vi "Acquire Data from Hardware N times.vi"(10 "User Specified":T1={"Hardware Configuration"={"Signal Channel"="PXI1Slot7/ao0", "Response Channel"="PXI1Slot7/ai0", "Trigger Channel"="/PXI1Slot7/PFI0", "Number of Acquisitions"=1.0}, "Analysis Configuration"={"Statistics"=TRUE}, "Signal Type"=enum."From Excel", "New Data Behavior"=enum."Replace", "Signal Configuration"={"Chirp Amplitude"=0.0, "I/O Limit"=0.0, "Sample Rate"=0.0, "Chirp Duration (s)"=0.0, "Upper Frequency"=0.0, "Lower Frequency"=0.0, "Windowing"=enum."None"}, "Waveform File"="", "Save Location"=""}) -> (0 "error out":errorcluster)   [LabVIEW 2017]
doc: "Generates sample waveforms according to the signal type in the HW Config input."
uses:
  controls/User Specified Data.ctl
  controls/HW Configuration.ctl
  controls/Analysis Configuration.ctl
  controls/New Data Behavior.ctl
  controls/Signal Configuration.ctl
  <vilib>/DAQmx/write.llb/DAQmx Write (Analog Wfm 1Chan NSamp).vi
  <vilib>/DAQmx/read.llb/DAQmx Read (Analog Wfm 1Chan NSamp).vi
  <vilib>/DAQmx/create/channels.llb/DAQmx Create Channel (AO-Voltage-Basic).vi
  <vilib>/DAQmx/configure/timing.llb/DAQmx Timing (Sample Clock).vi
  <vilib>/DAQmx/configure/trigger.llb/DAQmx Start Trigger (Digital Edge).vi
  <vilib>/DAQmx/miscellaneous.llb/DAQmx Fill In Error Info.vi
  <vilib>/DAQmx/create/channels.llb/DAQmx Create Channel (AI-Voltage-Basic).vi
  <vilib>/DAQmx/configure/task.llb/DAQmx Configure Logging (TDMS).vi
panel:
  in  "error in":errorcluster
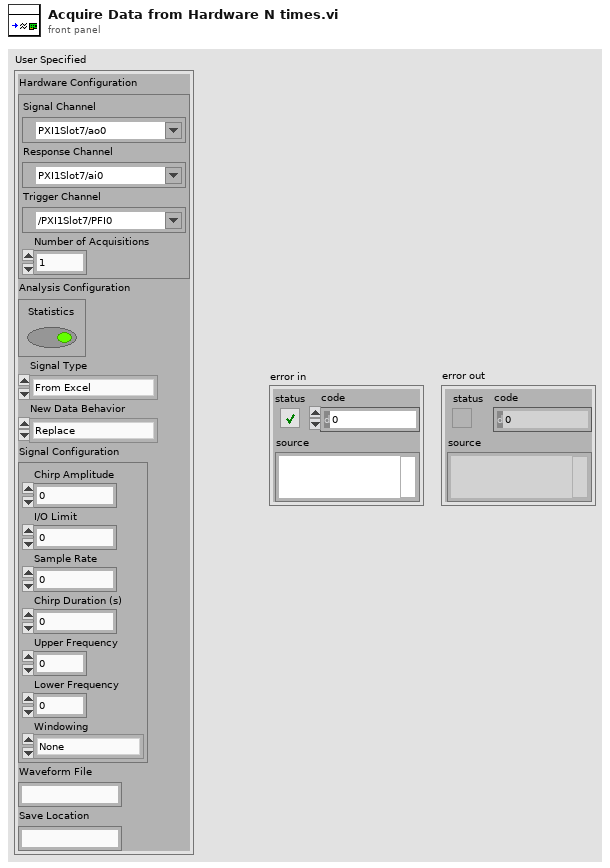
[diagram p1: front panel]
types:
  T1 = typedef "User Specified Data.ctl" = cluster{"Hardware Configuration":T2, "Analysis Configuration":T3, "Signal Type":enum16{"From Excel", "Single Chirp"}, "New Data Behavior":T4, "Signal Configuration":T5, "Waveform File":string, "Save Location":string}
  T2 = typedef "HW Configuration.ctl" = cluster{"Signal Channel":tag, "Response Channel":tag, "Trigger Channel":tag, "Number of Acquisitions":dbl}
  T3 = typedef "Analysis Configuration.ctl" = cluster{"Statistics":bool}
  T4 = typedef "New Data Behavior.ctl" = enum16{"Replace", "Overlay", "Append"}
  T5 = typedef "Signal Configuration.ctl" = cluster{"Chirp Amplitude":dbl, "I/O Limit":dbl, "Sample Rate":dbl, "Chirp Duration (s)":dbl, "Upper Frequency":dbl, "Lower Frequency":dbl, "Windowing":enum16{"None", "Exponential", "Flat top", "Hamming", "Hanning", "Kaiser-Bessel", "Rectangular"}}
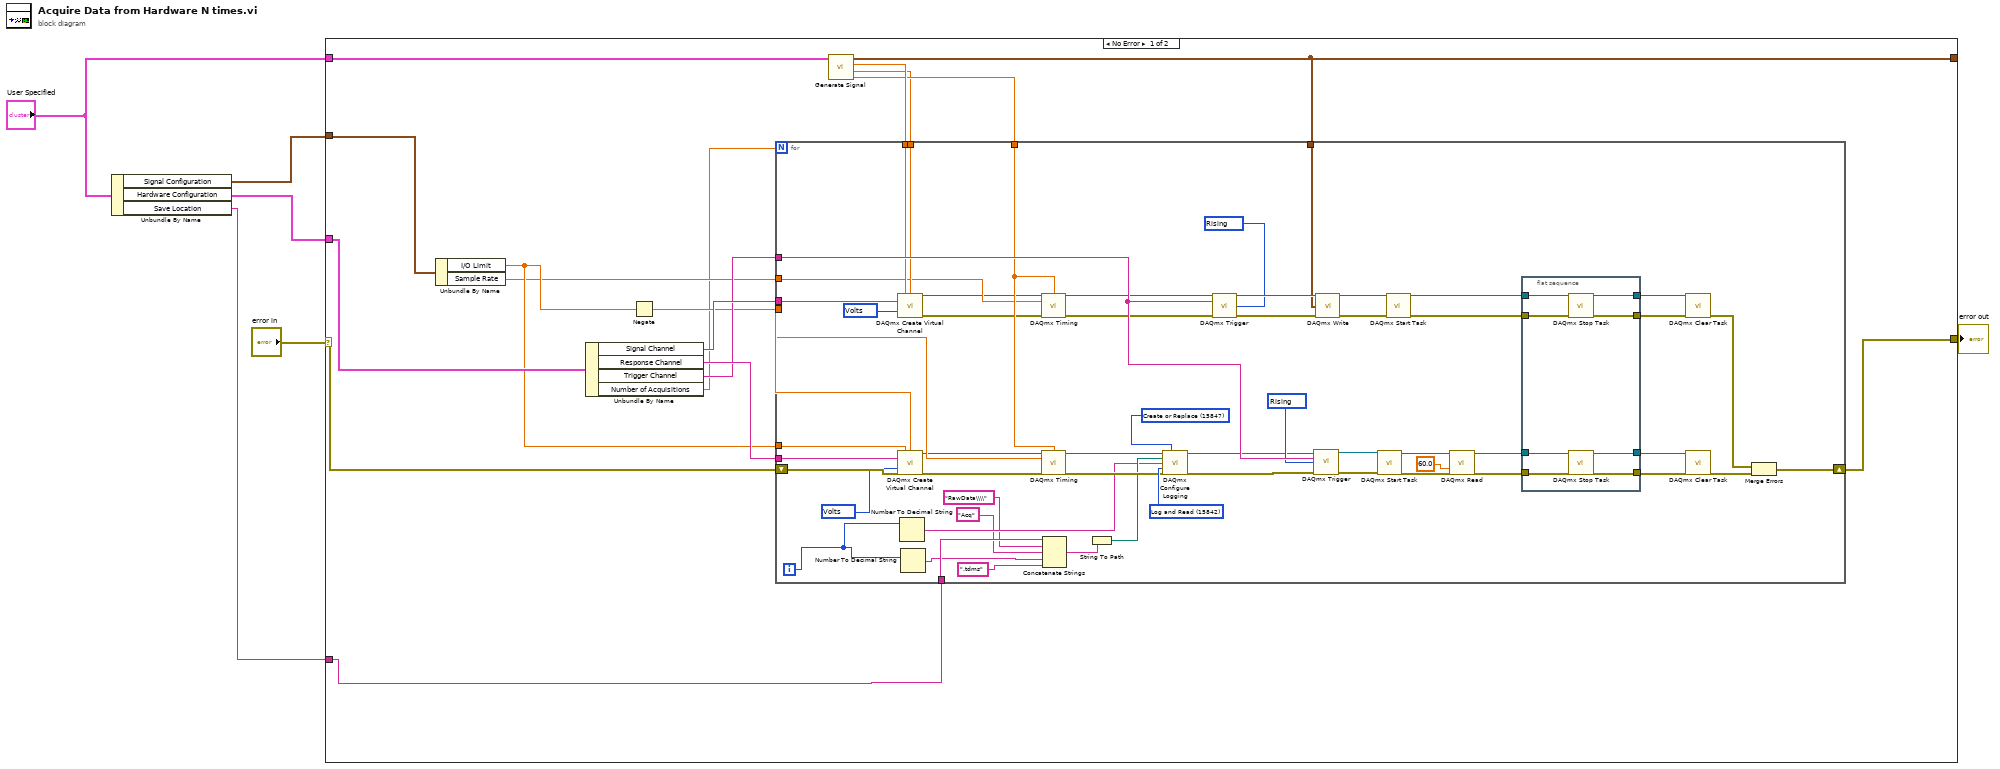
[diagram p0: block diagram]
diagram:
  n1 = Unbundle By Name("User Specified") -> ("Signal Configuration"=w4:T5, "Hardware Configuration"=w3:T2, "Save Location"=w2:string)
  n2 = case shown="No Error" "error in" {
    selector: "error in" -> [w22 w87]
    tunnel: w3 -> [w23 _]
    tunnel: [w19 w87] -> w6
    tunnel: [w9 _] -> _
    tunnel: w4 -> [w16 _]
    tunnel: "User Specified" -> [w14 _]
    tunnel: w2 -> [w7 _]
    frame No Error {
      n3 = Unbundle By Name(w16) -> ("I/O Limit"=w15:dbl, "Sample Rate"=w10:dbl)
      n4 = Unbundle By Name(w23) -> ("Signal Channel"=w20:tag, "Response Channel"=w21:tag, "Trigger Channel"=w18:tag, "Number of Acquisitions"=w8:dbl)
      n5 = Negate(x=w15) -> (-x=w17:dbl)
      n6 = call "Generate Signal.vi"("User Specified"=w14) -> ("Number of samples"=w12:dbl, "Y min"=w11:dbl, "Y max"=w13:dbl, "Final Waveform"=w9:waveform(dbl))  [unwired: 7 in]
      n7 = for {
        N: w8 -> [_]
        tunnel: w21 -> [w77]
        tunnel: w20 -> [w76]
        tunnel: w18 -> [w74]
        tunnel: w17 -> [w73]
        tunnel: w15 -> [w72]
        tunnel: w13 -> [w71]
        tunnel: w12 -> [w70]
        tunnel: w11 -> [w69]
        tunnel: w10 -> [w68]
        tunnel: w9 -> [w52]
        tunnel: w7 -> [w30]
        shift-right: [w75] -> w19
        shift-left: w22 -> [w78]
        i -> [w28]
        w44 = 15847 items=["Open"=10437, "Open or Create"=15846, "Create or Replace"=15847, "Create"=15848] ("operation")
        w45 = 15842 items=["Off"=10231, "Log"=15844, "Log and Read"=15842] ("logging mode")
        w48 = 10348 items=["Volts"=10348, "From Custom Scale"=10065] ("units")
        w49 = 10348 items=["Volts"=10348, "From Custom Scale"=10065] ("units")
        w54 = 10280 items=["Rising"=10280, "Falling"=10171] ("edge")
        w55 = 10280 items=["Rising"=10280, "Falling"=10171] ("edge")
        n8 = call-poly <vilib>:"DAQmx Create Virtual Channel.vi"("maximum value"=w71, "minimum value"=w69, "physical channels"=w76, "units"=w48) -> ("task out"=w63:refnum<k21>, "error out"=w62:errorcluster)  [unwired: 10 in]
        n9 = call-poly <vilib>:"DAQmx Create Virtual Channel.vi"("maximum value"=w72, "minimum value"=w73, "physical channels"=w77, "units"=w49, "error in"=w78) -> ("task out"=w64:refnum<k21>, "error out"=w65:errorcluster)  [unwired: 9 in]
        n10 = Number To Decimal String(number=w28) -> (decimal integer string=w29:string)  [unwired: 1 in]
        n11 = Number To Decimal String(number=w28) -> (decimal integer string=w24:string)  [unwired: 1 in]
        n12 = call-poly <vilib>:"DAQmx Timing.vi"("task/channels in"=w63, "samples per channel"=w70, "rate"=w68, "error in"=w62) -> ("task out"=w47:refnum<k21>, "error out"=w46:errorcluster)  [unwired: 10 in]
        n13 = call-poly <vilib>:"DAQmx Timing.vi"("task/channels in"=w64, "samples per channel"=w70, "rate"=w68, "error in"=w65) -> ("task out"=w41:refnum<k21>, "error out"=w40:errorcluster)  [unwired: 10 in]
        n14 = Concatenate Strings(w30, "RawData\\\\", "Acq", w24, ".tdms") -> (w32:string)
        n15 = String To Path(string=w32) -> (path=w31:path)
        n16 = call-poly <vilib>:"DAQmx Configure Logging.vi"("task/channels in"=w41, "operation"=w44, "file path"=w31, "group name"=w29, "logging mode"=w45, "error in"=w40) -> ("task out"=w43:refnum<k21>, "error out"=w42:errorcluster)  [unwired: 8 in]
        n17 = call-poly <vilib>:"DAQmx Trigger.vi"("task/channels in"=w47, "source"=w74, "edge"=w55, "error in"=w46) -> ("task out"=w56:refnum<k21>, "error out"=w57:errorcluster)  [unwired: 10 in]
        n18 = call-poly <vilib>:"DAQmx Trigger.vi"("task/channels in"=w43, "source"=w74, "edge"=w54, "error in"=w42) -> ("task out"=w39:refnum<k21>, "error out"=w38:errorcluster)  [unwired: 10 in]
        n19 = call-poly <vilib>:"DAQmx Write.vi"("task/channels in"=w56, "data"=w52) -> ("task out"=w53:refnum<k21>)  [unwired: 11 in, 2 out]
        n20 = call <vilib>:"DAQmx Start Task.vi"("task/channels in"=w39, "error in"=w38) -> ("task out"=w36:refnum<k21>, "error out"=w35:errorcluster)  [unwired: 12 in]
        n21 = call <vilib>:"DAQmx Start Task.vi"("task/channels in"=w53, "error in"=w57) -> ("task out"=w50:refnum<k21>, "error out"=w51:errorcluster)  [unwired: 12 in]
        n22 = call-poly <vilib>:"DAQmx Read.vi"("task/channels in"=w36, "timeout"=60.0, "error in"=w35) -> ("task out"=w34:refnum<k21>, "error out"=w33:errorcluster)  [unwired: 10 in, 1 out]
        n23 = flat-sequence {
          tunnel: [w86] -> w67
          tunnel: [w85] -> w66
          tunnel: [w84] -> w60
          tunnel: [w83] -> w58
          tunnel: w34 -> [w82]
          tunnel: w33 -> [w81]
          tunnel: w51 -> [w80]
          tunnel: w50 -> [w79]
          frame #0 {
            n24 = call <vilib>:"DAQmx Stop Task.vi"("task/channels in"=w79, "error in"=w80) -> ("task out"=w83:refnum<k21>, "error out"=w84:errorcluster)  [unwired: 12 in]
            n25 = call <vilib>:"DAQmx Stop Task.vi"("task/channels in"=w82, "error in"=w81) -> ("task out"=w85:refnum<k21>, "error out"=w86:errorcluster)  [unwired: 12 in]
          }
        }
        n26 = call <vilib>:"DAQmx Clear Task.vi"("task in"=w58, "error in"=w60) -> ("error out"=w59:errorcluster)  [unwired: 13 in]
        n27 = call <vilib>:"DAQmx Clear Task.vi"("task in"=w66, "error in"=w67) -> ("error out"=w61:errorcluster)  [unwired: 13 in]
        n28 = Merge Errors(w59, w61) -> (w75:errorcluster)
      }
    }
    frame Error {
    }
  }
  "error out" <- w6
